vi "GetCases.vi"(6 "error in":errorcluster, 9 "CaseStructure in":refnum<class "CaseStructure.lvclass">) -> (0 "error out":errorcluster, 3 "CaseStructure out":refnum<class "CaseStructure.lvclass">, 4 "cases":string, 5 "diagram indices":i32[](array[numeric]))   [LabVIEW 2014, in "CaseStructure.lvclass"]
uses:
  CaseStructure.lvclass
  Python/Parsing/ListTypesTD.ctl
  <vilib>/Utility/VariantDataType/VariantType.lvlib
  Python/Parsing/Python Functions.lvlib
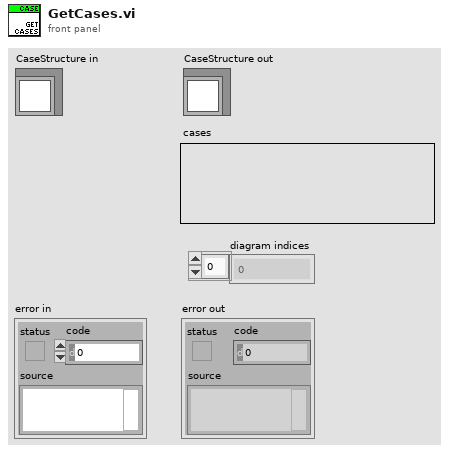
[diagram p1: front panel]
types:
  T1 = typedef "Python Functions.lvlib/ListTypesTD.ctl" = enum16{"list", "tuple", "parameter list", "output list", "return values"}
  T2 = typedef "VariantType.lvlib/Type.ctl" = enum8{"Invalid Type", "Void", "I8", "I16", "I32", "I64", "U8", "U16", "U32", "U64", "Single Float", "Double Float", "Extended Float", "Single Complex", "Double Complex", "Extended Complex", "Enum U8", "Enum U16", "Enum U32", "Enum U64", "Single Float With Unit", "Double Float With Unit", "Extended Float With Unit", "Single Complex with Unit", "Double Complex with Unit", "Extended Complex with Unit", "Boolean", "String", "Path", "Picture", "Tag", "Array", "Cluster", "Variant", "LV Variant", "Waveform", "Timestamp", "Digital Waveform", "Digital Data", "ExpressData", "Refnum", "External Data", "VI", "Poly VI", "LabVIEW Class Instance", "Fixed Point"}
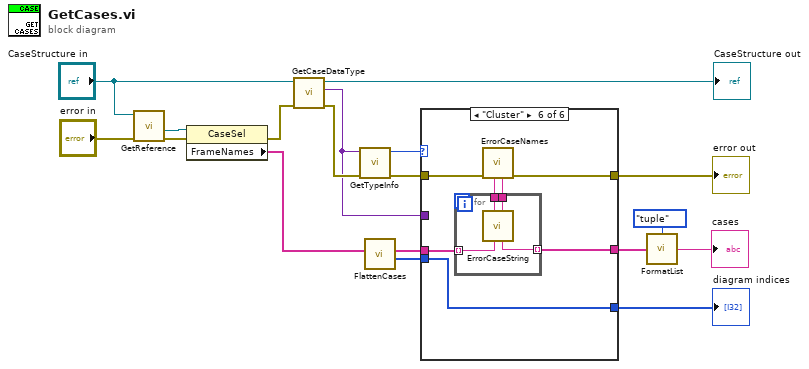
[diagram p0: block diagram]
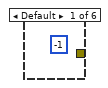
[diagram p2: hidden frame]
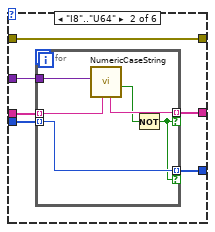
[diagram p3: hidden frame]
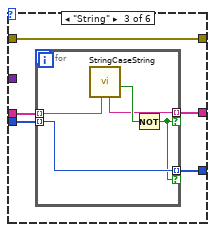
[diagram p4: hidden frame]
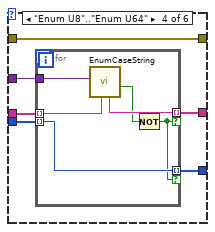
[diagram p5: hidden frame]
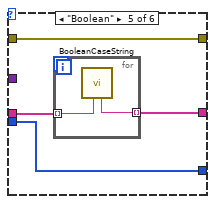
[diagram p6: hidden frame]
diagram:
  n1 = call "GetReference.vi"("error in"="error in", "CaseStructure in"="CaseStructure in") -> ("error out"=w17:errorcluster, "reference out"=w18:refnum<vi>)  [unwired: 7 in, 1 out]
  n2 = property class="CaseSel"(reference=w18, error in=w17) -> (error out=w14:errorcluster, "FrameNames"=w4:string[])  [unwired: 1 out]
  n3 = call "GetCaseDataType.vi"("error in"=w14, "CaseStructure in"="CaseStructure in") -> ("error out"=w12:errorcluster, "Data Type"=w5:variant, "CaseStructure out"=→"CaseStructure out":refnum<class "CaseStructure.lvclass">)  [unwired: 5 in]
  n4 = call <vilib>:"GetTypeInfo.vi"("error in (no error)"=w12, "Variant"=w5) -> ("error out"=w10:errorcluster, "Type Enum"=w11:T2)  [unwired: 5 in, 3 out]
  n5 = call "FlattenCases.vi"("Frame Names"=w4) -> ("diagram index"=w2:i32[], "cases"=w3:string[])  [unwired: 9 in]
  n6 = case shown="\"Cluster\"" w11 {
    tunnel: w10 -> [_ w22 w33 w44 w54 w62]
    tunnel: w3 -> [_ w24 w35 w46 w56 w65]
    tunnel: [_ w23 w34 w45 w53 w63] -> w8
    tunnel: [_ w22 w33 w44 w54 w61] -> w6
    tunnel: w5 -> [_ w21 _ w41 _ _]
    tunnel: w2 -> [_ w20 w32 w43 w55 w64]
    tunnel: [_ w19 w31 w42 w55 w64] -> w1
    frame Default {
      (unwired) -1
    }
    frame "I8".."U64" {
      n7 = for {
        tunnel: w24 -> [w30] mode=indexing
        tunnel: [w29] -> w23 mode=indexing if=w25
        tunnel: w21 -> [w27]
        tunnel: w20 -> [w26] mode=indexing
        tunnel: [w26] -> w19 mode=indexing if=w25
        n8 = call "NumericCaseString.vi"("selector string"=w30, "data type"=w27) -> ("Default"=w28:bool, "case"=w29:string)  [unwired: 6 in]
        n9 = Not(x=w28) -> (.not. x?=w25:bool)
      }
    }
    frame "String" {
      n10 = for {
        tunnel: w35 -> [w36] mode=indexing
        tunnel: [w37] -> w34 mode=indexing if=w39
        tunnel: w32 -> [w40] mode=indexing
        tunnel: [w40] -> w31 mode=indexing if=w39
        n11 = call "StringCaseString.vi"("selector string"=w36) -> ("Default"=w38:bool, "case"=w37:string)  [unwired: 7 in]
        n12 = Not(x=w38) -> (.not. x?=w39:bool)
      }
    }
    frame "Enum U8".."Enum U64" {
      n13 = for {
        tunnel: w46 -> [w50] mode=indexing
        tunnel: [w49] -> w45 mode=indexing if=w51
        tunnel: w43 -> [w52] mode=indexing
        tunnel: [w52] -> w42 mode=indexing if=w51
        tunnel: w41 -> [w47]
        n14 = call "EnumCaseString.vi"("selector string"=w50, "data type"=w47) -> ("Default"=w48:bool, "case"=w49:string)  [unwired: 6 in]
        n15 = Not(x=w48) -> (.not. x?=w51:bool)
      }
    }
    frame "Boolean" {
      n16 = for {
        tunnel: w56 -> [w58] mode=indexing
        tunnel: [w57] -> w53 mode=indexing
        n17 = call "BooleanCaseString.vi"("selector string"=w58) -> ("case"=w57:string)  [unwired: 7 in, 1 out]
      }
    }
    frame "Cluster" {
      n18 = call "ErrorCaseNames.vi"("error in"=w62) -> ("error out"=w61:errorcluster, "Error"=w59:string, "No Error"=w60:string)  [unwired: 6 in]
      n19 = for {
        tunnel: w65 -> [w69] mode=indexing
        tunnel: [w68] -> w63 mode=indexing
        tunnel: w60 -> [w67]
        tunnel: w59 -> [w66]
        n20 = call "ErrorCaseString.vi"("Error"=w66, "selector string"=w69, "No Error"=w67) -> ("case"=w68:string)  [unwired: 7 in, 1 out]
      }
    }
  }
  "error out" <- w6
  "diagram indices" <- w1
  n21 = call "FormatList.vi"("values"=w8, "type"=ListTypesTD."tuple") -> ("python object"=→"cases":string)
